vi "P-541 Wait for Move.vi"(0 "VISA Ref":refnum<visa-resource-name>, 2 "Threshold":dbl=0.003, 7 "Axis Name":string, 11 "Error In":errorcluster) -> (4 "VISA Ref Dup":refnum<visa-resource-name>, 8 "Position":dbl, 15 "Error Out":errorcluster)   [LabVIEW 2020]
panel:
  out "Position vs Time":dbl[](graph)
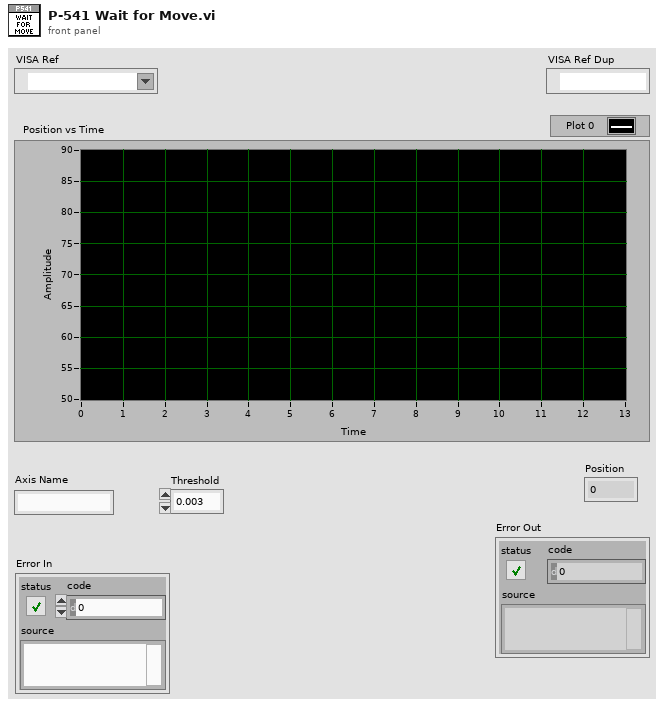
[diagram p1: front panel]
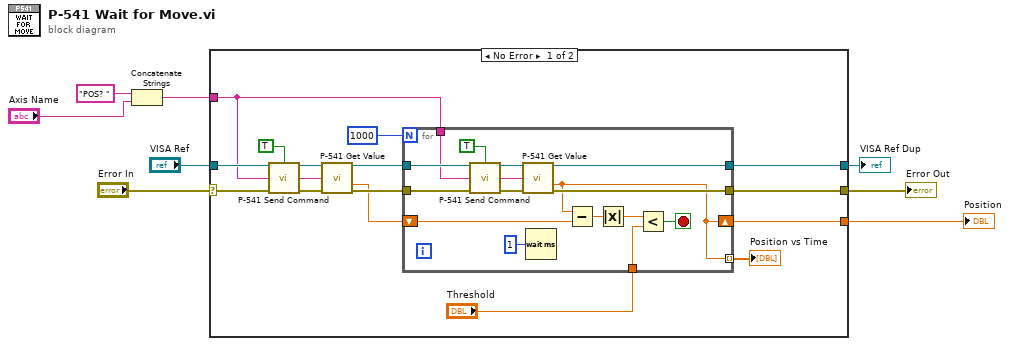
[diagram p0: block diagram]
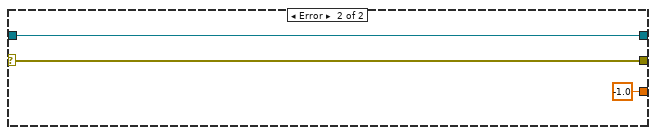
[diagram p2: hidden frame]
diagram:
  n1 = Concatenate Strings("POS? ", "Axis Name") -> (w1:string)
  n2 = case shown="No Error" "Error In" {
    selector: "Error In" -> [w15 w42]
    tunnel: "VISA Ref" -> [w16 w43]
    tunnel: [w12 w43] -> w6
    tunnel: [w11 w42] -> w5
    tunnel: [w10 -1.0 ("Value")] -> w4
    tunnel: w1 -> [w9 _]
    frame No Error {
      n3 = call "P-541 Send Command.vi"("VISA Ref"=w16, "Wait for Reply (T)"=TRUE, "Command"=w9, "Error In"=w15) -> ("VISA Ref Dup"=w22:refnum<visa-resource-name>, "Reply"=w23:string, "Error Out"=w24:errorcluster)  [unwired: 8 in, 1 out]
      n4 = call "P-541 Get Value.vi"("VISA Pass Thru"=w22, "Cmd Reply"=w23, "Error In"=w24) -> ("VISA Ref Dup"=w20:refnum<visa-resource-name>, "Value"=w18:dbl, "Error Out"=w19:errorcluster)  [unwired: 9 in, 1 out]
      n5 = for {
        N: 1000 -> [_]
        tunnel: w20 -> [w39]
        tunnel: w19 -> [w38]
        shift-right: [w25] -> w10
        shift-left: w18 -> [w34]
        tunnel: [w32] -> w12
        tunnel: [w28] -> w11
        tunnel: w9 -> [w27]
        tunnel: "Threshold" -> [w26]
        tunnel: [w25] -> w13 mode=indexing
        stop <- w30 stop-if-true
        n6 = call "P-541 Send Command.vi"("VISA Ref"=w39, "Wait for Reply (T)"=TRUE, "Command"=w27, "Error In"=w38) -> ("VISA Ref Dup"=w37:refnum<visa-resource-name>, "Reply"=w36:string, "Error Out"=w35:errorcluster)  [unwired: 8 in, 1 out]
        n7 = call "P-541 Get Value.vi"("VISA Pass Thru"=w37, "Cmd Reply"=w36, "Error In"=w35) -> ("VISA Ref Dup"=w32:refnum<visa-resource-name>, "Value"=w25:dbl, "Error Out"=w28:errorcluster)  [unwired: 9 in, 1 out]
        n8 = Wait (ms)(milliseconds to wait=u32 1) -> ()  [unwired: 1 out]
        n9 = Subtract(x=w25, y=w34) -> (x-y=w33:dbl)
        n10 = Absolute Value(x=w33) -> (abs(x)=w31:dbl)
        n11 = Less?(x=w31, y=w26) -> (x < y?=w30:bool)
      }
      "Position vs Time" <- w13
    }
    frame Error {
    }
  }
  "Error Out" <- w5
  "VISA Ref Dup" <- w6
  "Position" <- w4
